vi "get_data_folder_path.vi"(8 "error in (no error)":errorcluster) -> (0 "error out":errorcluster, 2 "data folder path":path)   [LabVIEW 2010]
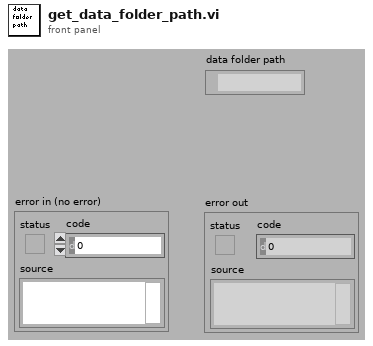
[diagram p1: front panel]
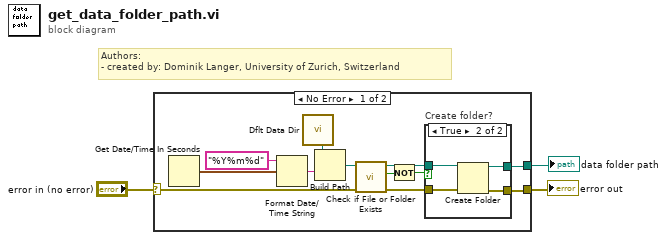
[diagram p0: block diagram]
diagram:
  # "Authors: \n- created by: Dominik Langer, University of Zurich, Switzerland"
  n1 = case shown="No Error" "error in (no error)" {
    selector: "error in (no error)" -> [w10 w22]
    tunnel: [w6 w22] -> w2
    tunnel: [w4 _] -> w1
    frame No Error {
      n2 = Get Date/Time In Seconds() -> (seconds since 1Jan1904=w15:timestamp)
      n3 = Format Date/Time String(time format string (%c)="%Y%m%d", seconds (now)=w15) -> (date/time string=w13:string)  [unwired: 1 out]
      n4 = call <vilib>:"Dflt Data Dir.vi"() -> ("App:Default Data Directory"=w12:path)
      n5 = Build Path(base path=w12, name or relative path=w13) -> (appended path=w11:path)
      n6 = call <vilib>:"Check if File or Folder Exists.vi"("error in (no error)"=w10, "path"=w11) -> ("error out"=w9:errorcluster, "file or folder exists?"=w8:bool, "dup path"=w5:path)  [unwired: 7 out]
      n7 = Not(x=w8) -> (.not. x?=w7:bool)
      n8 = case "Create folder?" shown="True" w7 {
        tunnel: w9 -> [w17 w21]
        tunnel: [w17 w20] -> w6
        tunnel: w5 -> [w16 w19]
        tunnel: [w16 w18] -> w4
        frame False {
        }
        frame True {
          n9 = Create Folder(path (use dialog)=w19, error in=w21) -> (created path=w18:path, error out=w20:errorcluster)  [unwired: 2 out]
        }
      }
    }
    frame Error {
    }
  }
  "error out" <- w2
  "data folder path" <- w1
